vi "ArmRawToLimitedRLE.vi"(9 "rawE":dbl, 10 "rawL":dbl, 11 "rawR":dbl) -> (1 "limE":dbl, 2 "limL":dbl, 3 "limR":dbl)   [LabVIEW 2020]
doc: "inputs raw RLE, outputs limited RLE\n\ninputs\n --raw RLE -- Double\n\noutputs\n --limited RLE -- Double"
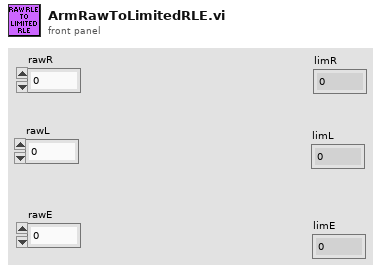
[diagram p1: front panel]
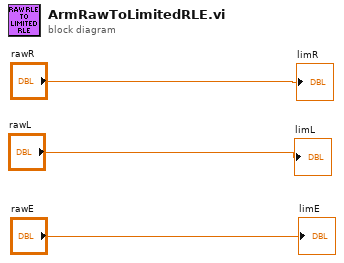
[diagram p0: block diagram]
diagram:
  "limR" <- "rawR"
  "limL" <- "rawL"
  "limE" <- "rawE"
